vi "test Receive Connected Messages.vi"(8 "error in (no error)":errorcluster, 11 "TestCase in":refnum<class "Test Nested Endpoint Transmit Failure.lvclass">) -> (0 "error out":errorcluster, 3 "TestCase out":refnum<class "Test Nested Endpoint Transmit Failure.lvclass">)   [LabVIEW 2014]
uses:
  <vilib>/addons/_JKI Toolkits/VI Tester/TestCase.llb/TestCase.lvclass
  <vilib>/ActorFramework/Message Queue/Message Queue.lvclass
  Test Nested Endpoint Transmit Failure.lvclass
  <vilib>/ActorFramework/Message Dequeuer/Message Dequeuer.lvclass
  <vilib>/ActorFramework/Message Enqueuer/Message Enqueuer.lvclass
  Nested Endpoint/Nested Endpoint Messages/Connected Msg/Connected Msg.lvclass
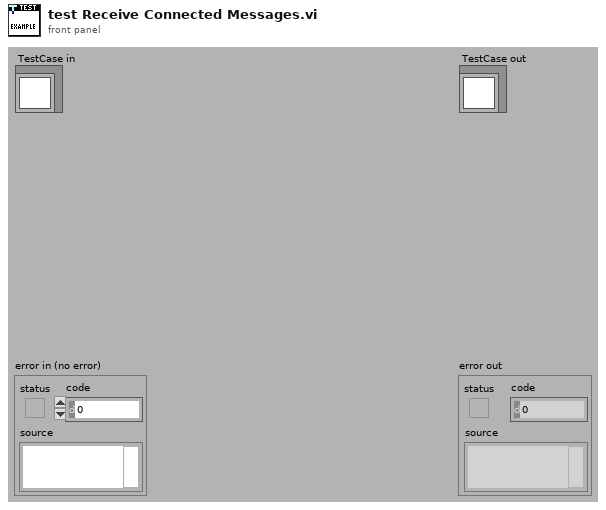
[diagram p1: front panel]
types:
  T1 = cluster{"Endpoint Enqueuer":refnum<class "Message Enqueuer.lvclass">}
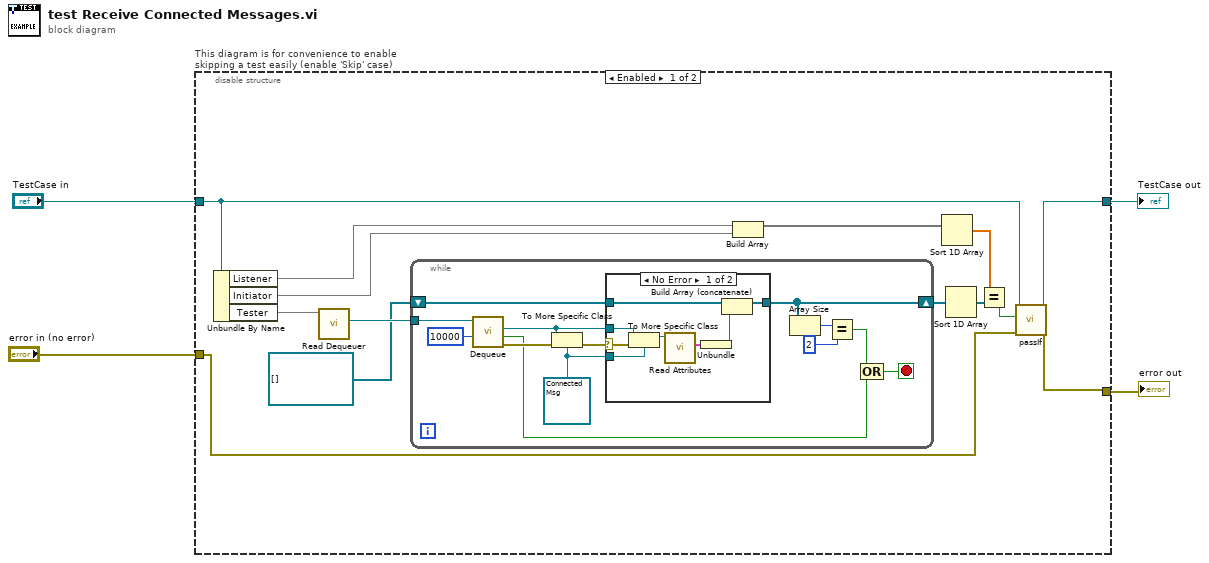
[diagram p0: block diagram]
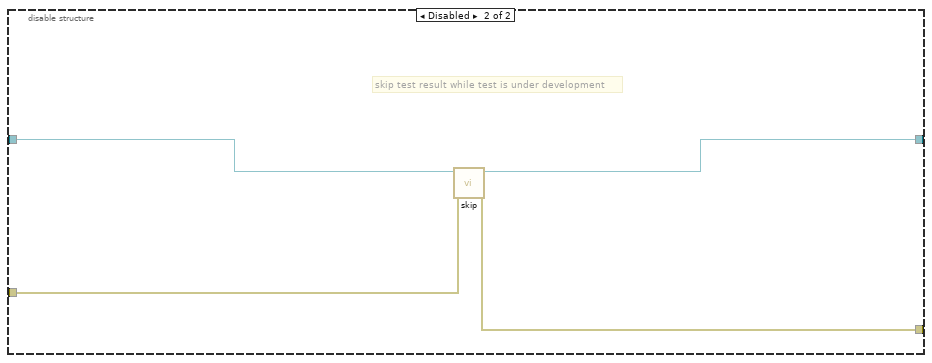
[diagram p3: hidden frame]
diagram:
  n1 = disable-structure "This diagram is for convenience to enable skipping a test easily (enable 'Skip' case)" shown="Enabled" {
    disable-tunnel: "TestCase in" -> [w16 w44]
    disable-tunnel: [w18 w42] -> w1
    disable-tunnel: [w17 w43] -> w3
    disable-tunnel: "error in (no error)" -> [w14 w41]
    frame Enabled {
      n2 = Unbundle By Name(w16) -> ("Listener"=w8, "Initiator"=w9, "Tester"=w15)
      n3 = call <vilib>:"Read Dequeuer.vi"("Message Queue"=w15) -> ("Message Dequeuer"=w13:refnum<class "Message Dequeuer.lvclass">)  [unwired: 10 in]
      n4 = while {
        tunnel: w13 -> [w31]
        shift-right: [w22] -> w11
        shift-left: refnum<class "Message Enqueuer.lvclass">[] [] -> [w23]
        stop <- w28 stop-if-true
        w24 = refnum<class "Connected Msg.lvclass"> refnum ("Nested Endpoint.lvlib:Connected Msg.lvclass")
        n5 = call <vilib>:"Dequeue.vi"("timeout in ms (-1)"=10000, "Message Dequeuer in"=w31) -> ("error out"=w29:errorcluster, "timed out?"=w27:bool, "Message"=w25:refnum<class "Message.lvclass">)  [unwired: 5 in, 2 out]
        n6 = To More Specific Class(target class=w24, reference=w25, error in=w29) -> (error out=w26:errorcluster)  [unwired: 1 out]
        n7 = case shown="No Error" w26 {
          selector: w26 -> [w39 _]
          tunnel: w25 -> [w38 _]
          tunnel: w24 -> [w37 _]
          tunnel: w23 -> [w34 w40]
          tunnel: [w33 w40] -> w22
          frame No Error {
            n8 = To More Specific Class(target class=w37, reference=w38, error in=w39) -> (specific class reference=w36:refnum<class "Connected Msg.lvclass">)  [unwired: 1 out]
            n9 = call "Read Attributes.vi"("Connected Msg"=w36) -> ("Payload"=w35:T1)  [unwired: 10 in]
            n10 = Unbundle(w35) -> ("Endpoint Enqueuer"=w32:refnum<class "Message Enqueuer.lvclass">)
            n11 = Build Array (concatenate)(w34, w32) -> (w33:refnum<class "Message Enqueuer.lvclass">[])
          }
          frame Error {
          }
        }
        n12 = Array Size(array=w22) -> (size(s)=w21:i32)
        n13 = Equal?(x=w21, y=2) -> (x = y?=w19:bool)
        n14 = Compound Arithmetic op=OR(w19, w27) -> (w28:bool)
      }
      n15 = Build Array(w8, w9) -> (w7:void[])
      n16 = Sort 1D Array(array=w7) -> (sorted array=w6:dbl[])
      n17 = Sort 1D Array(array=w11) -> (sorted array=w10:refnum<class "Message Enqueuer.lvclass">[])
      n18 = Equal?(x=w6, y=w10) -> (x = y?=w5:bool)
      n19 = call-dynamic "passIf.vi"("error in (no error)"=w14, "pass"=w5, "TestCase in"=w16) -> ("error out"=w17:errorcluster, "TestCase out"=w18:refnum<class "Test Nested Endpoint Transmit Failure.lvclass">)  [unwired: 7 in]
    }
    frame Disabled {
      # "skip test result while test is under development"
      n20 = call <vilib>:"skip.vi"("error in (no error)"=w41, "TestCase in"=w44) -> ("error out"=w43:errorcluster, "TestCase out"=w42:refnum<class "Test Nested Endpoint Transmit Failure.lvclass">)  [unwired: 8 in]
    }
  }
  "error out" <- w3
  "TestCase out" <- w1
